vi "ClassPanel.vi"(8 "error in (no error)":errorcluster caption="entrée d'erreur (pas d'erreur)", 11 "DAQ6363.lvclass":refnum<class "DAQ6363.lvclass">) -> (0 "error out":errorcluster caption="sortie d'erreur", 3 "DAQ6363.lvclass Out":refnum<class "DAQ6363.lvclass">)   [LabVIEW 2019, in "DAQ6363.lvclass"]
uses:
  DAQ6363.lvclass
  C:/Programmes Labview/LabScanV1A/DevicesClass/BaseDevice/BaseDevice.lvclass
  BaseDevice/ClassQueueMess.ctl
  BaseDevice/BaseDevice.lvclass/BaseDevice.ctl
  DAQ6363.lvclass/DAQ6363.ctl
  BaseDevice/Accessor/SetShowInstrNm.vi
  BaseDevice/Accessor/GetClassEvent.vi
  <vilib>/DAQmx/create/channels.llb/DAQmx Create Channel (CI-Count Edges).vi
  <resource>/objmgr/daqmx.rc
panel:
  out "RtAvg Data":i32[][](array[numeric]) format="%.2f"
  out "Rate Data":i32[][](array[numeric])
  out "ClearRef":refnum<vi>
  out "Graph":refnum<vi>
  out "Dat":refnum<vi>
  out "ViRef":refnum<vi>
  out "Avg ref":refnum<vi>
  out "RtGrphAct":bool
  out "DeltaCh2(ms)":u32
  out "DeltaCh1(ms)":u32
  out "ReadCnts":bool
  out "Ch2CntTask":refnum<k21>
  out "Ch1CntTask":refnum<k21>
  in  "DAQ6363 Tabs":enum32{"Main", "Advanced"}(tab)
  in  "AcqTime":dbl=60.0 caption="Acqu. Time (ms)" min=0.1 step=0.1 format="%#.1f"
  out "TimeLeft":dbl caption="Time left(ms)" format="%<%H:%M:%S%1u>t"
  in  "ReadCont":bool caption="Read\nCont."
  out "Count Rates":u32[](array[numeric]) format="%#.0f"
  in  "ClearGrp":bool
  in  "Rate Graph":bool caption="Rate\nGraph"
  in  "Channel 1":bool
  in  "Channel 2":bool
  out "Jitter":bool
  in  "edge 2":i32(ring)=10280 caption="Ch2 Edge" items=["Rising"=10280, "Falling"=10171]
  in  "Ch2 Counter":tag="Dev1/ctr1"
  in  "Ch1 Counter":tag="Dev1/ctr0"
  in  "edge":i32(ring)=10280 caption="Ch1 Edge" items=["Rising"=10280, "Falling"=10171]
  in  "Ch1 Input":tag="/Dev1/PFI10"
  in  "Ch2 Input":tag="PFI8"
  in  "MainProgQ":refnum<queue>
  in  "MainProgQEvent":refnum<user-event>
  in  "Acq":bool
  in  "Stop":bool
  out "Init Program":bool
  # "DAQ6363"
  # "this MUST labeled with class name"
  # "this MUST be present and labeled \"Stop\" and \"Acq\""
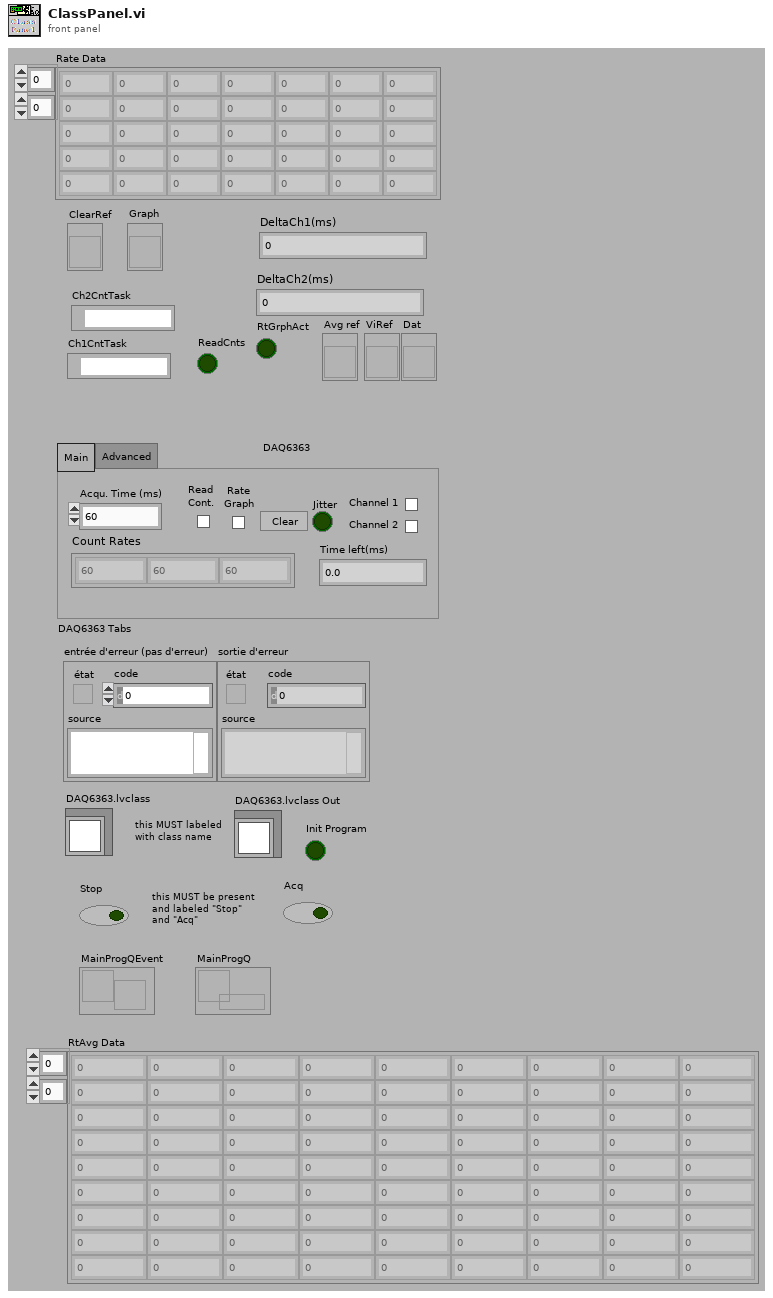
[diagram p1: front panel]
types:
  T1 = enum32{"Invalid", "Standard", "Closed", "Hidden", "Minimized", "Maximized"}
  T2 = cluster{dbl, "Refresh(ms)":u32, "Rate Data Out":i32[][]}
  T3 = typedef "ClassQueueMess.ctl" = u16
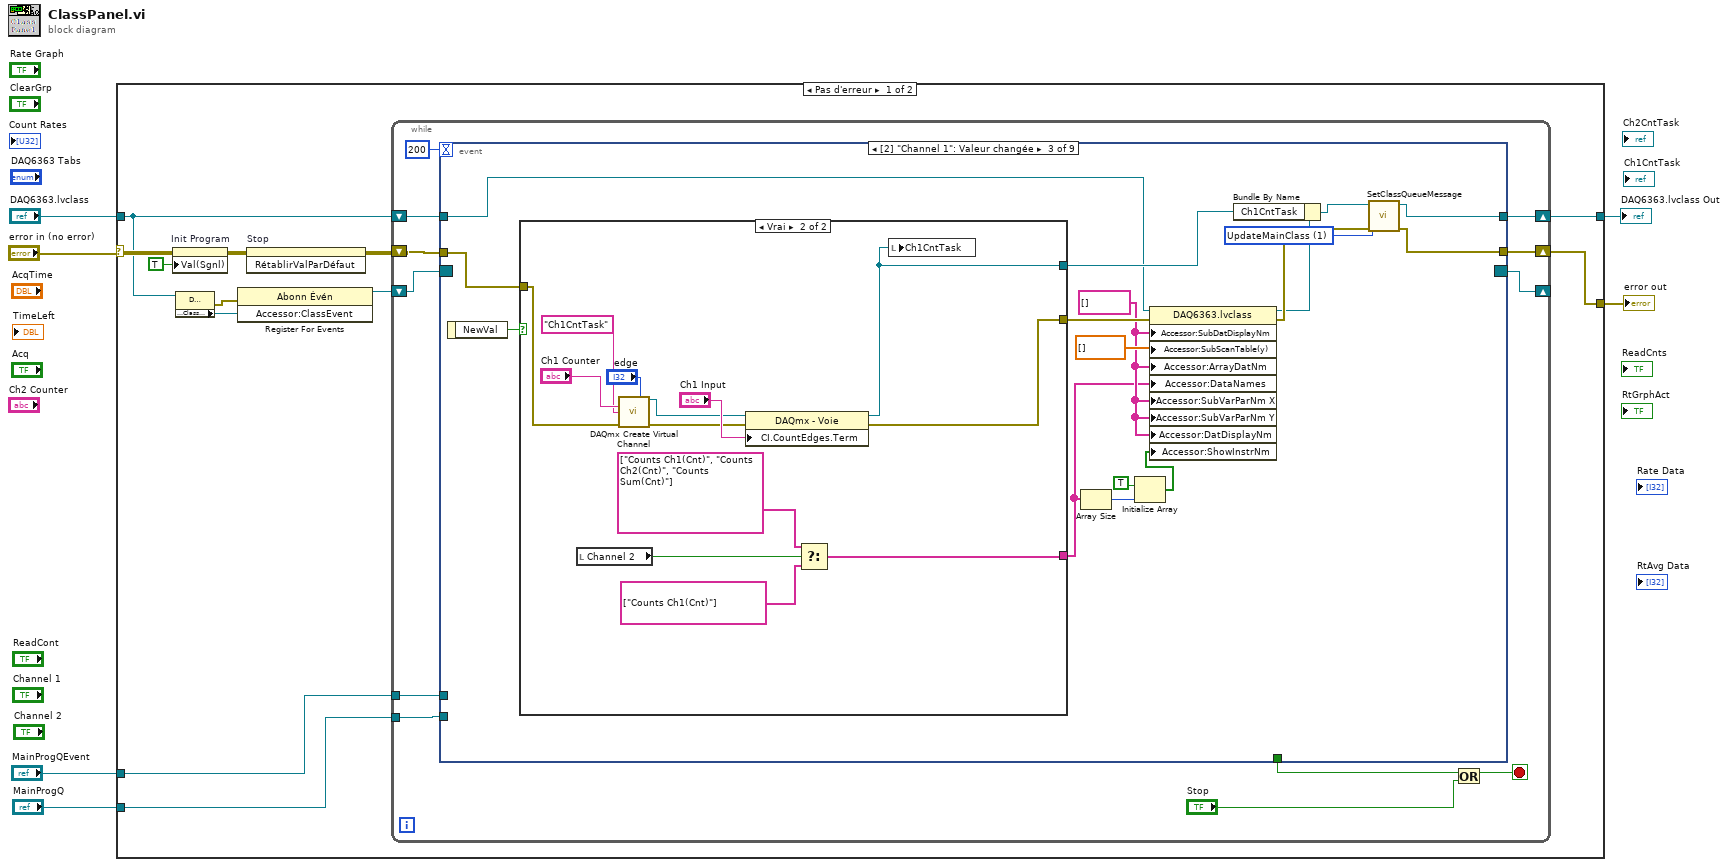
[diagram p0: block diagram]
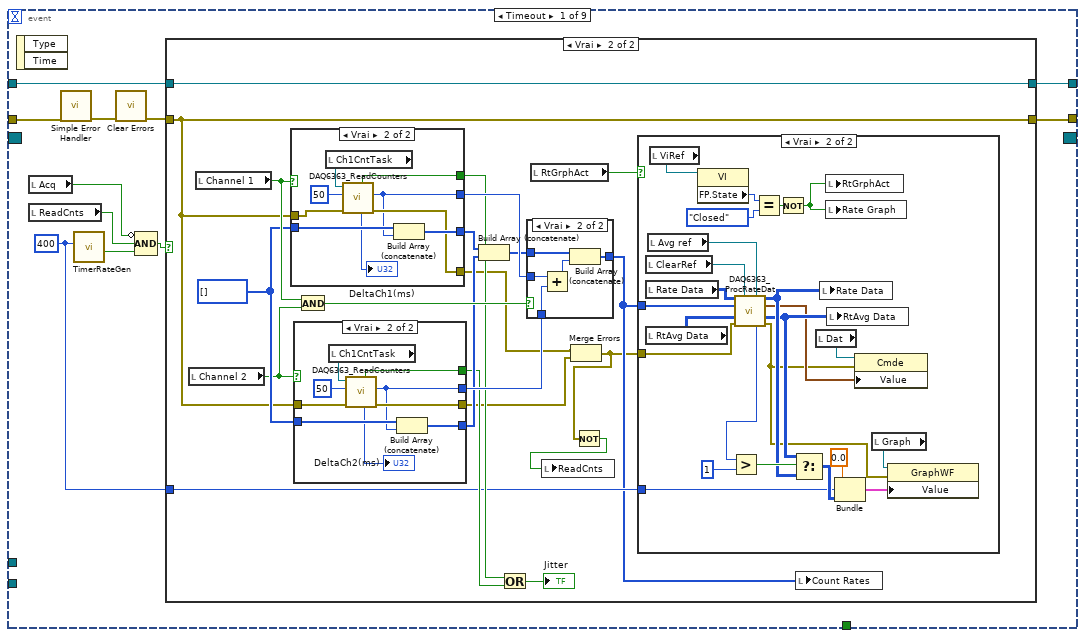
[diagram p2: hidden frame]
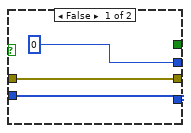
[diagram p5: hidden frame]
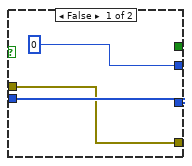
[diagram p7: hidden frame]
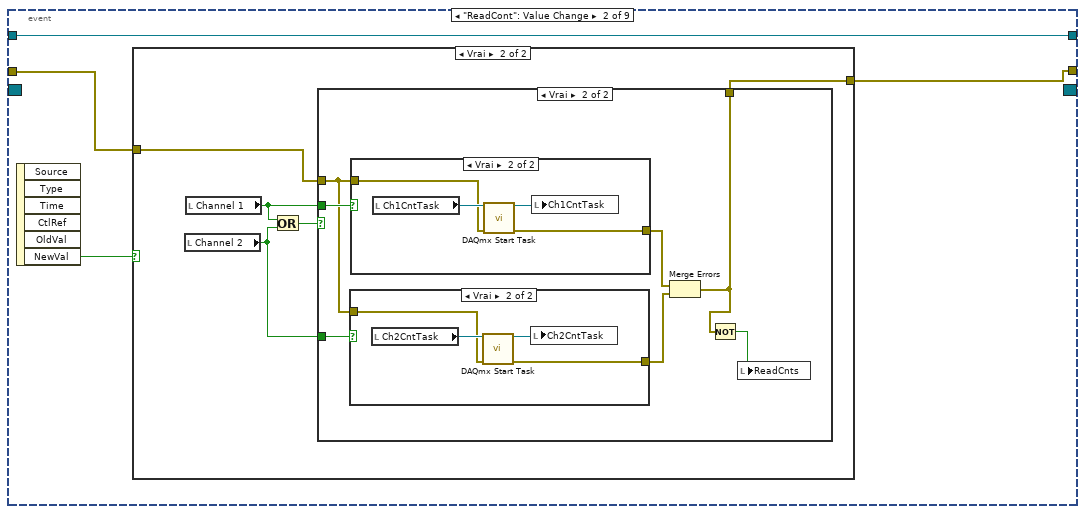
[diagram p8: hidden frame]
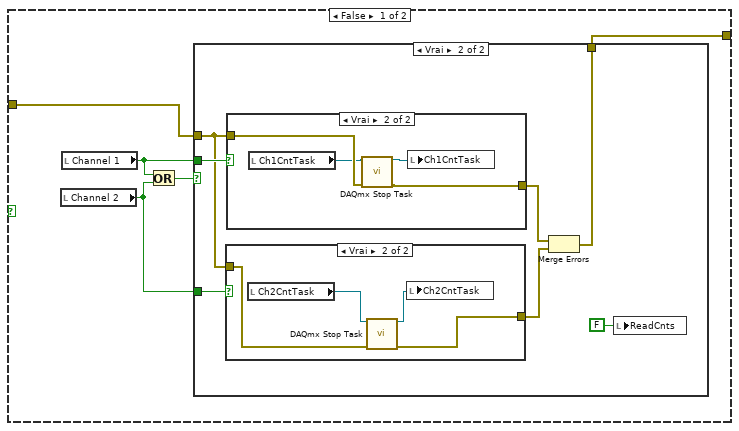
[diagram p9: hidden frame]
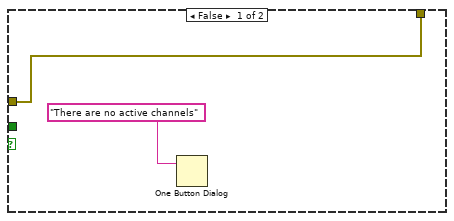
[diagram p13: hidden frame]
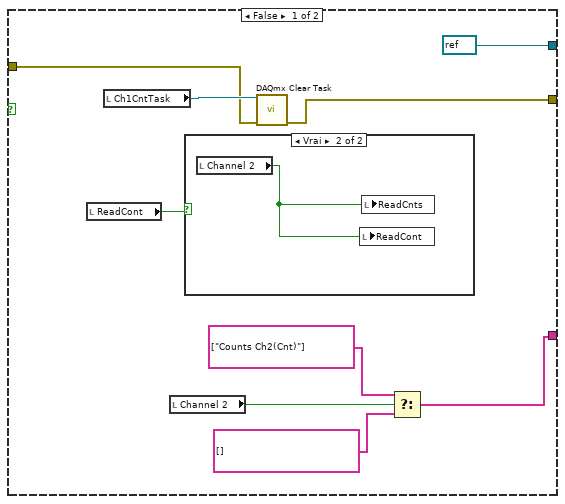
[diagram p16: hidden frame]
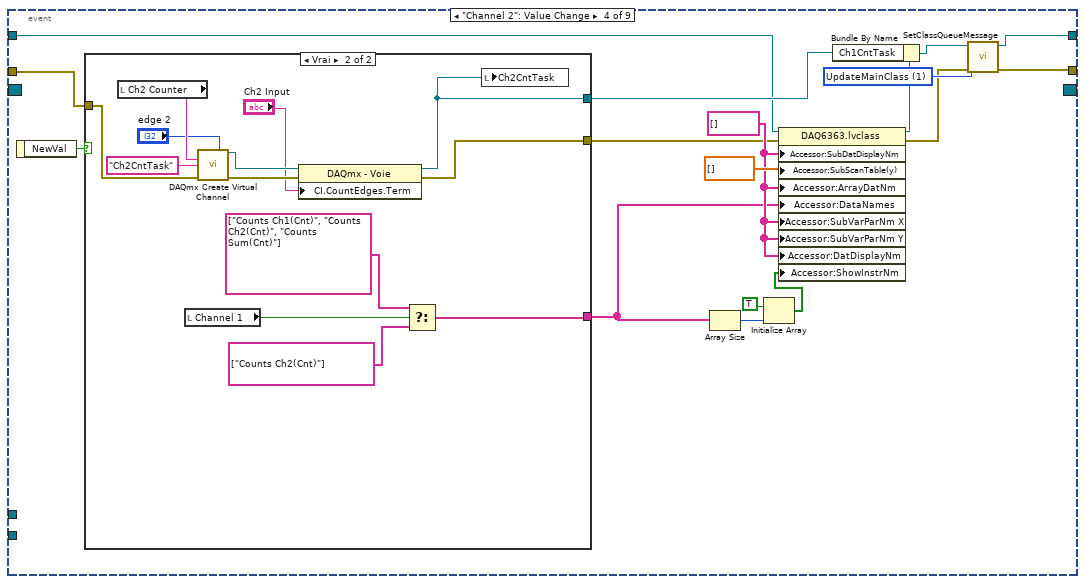
[diagram p18: hidden frame]
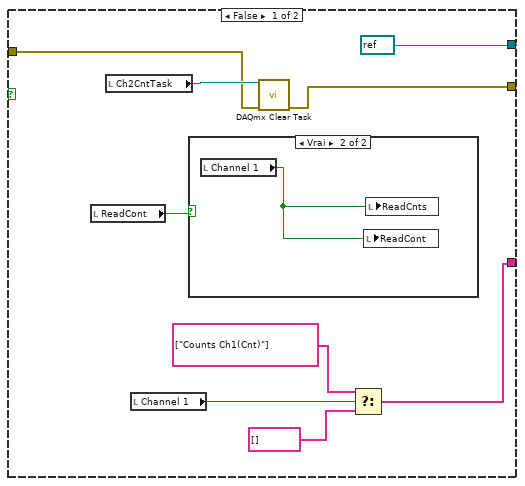
[diagram p19: hidden frame]
diagram:
  n1 = case shown="Pas d'erreur" "error in (no error)" {
    selector: "error in (no error)" -> [w15 w329]
    tunnel: [w18 w329] -> w5
    tunnel: "DAQ6363.lvclass" -> [w10 w328]
    tunnel: [w16 w328] -> w3
    tunnel: "MainProgQEvent" -> [w8 _]
    tunnel: "MainProgQ" -> [w7 _]
    frame No Error {
      n2 = property on="Init Program" class="Bool (strict)"(error in=w15, "Val(Sgnl)"=TRUE ("Valeur (Signalisation)")) -> (error out=w14:errorcluster)  [unwired: 1 in, 1 out]
      n3 = property class="DAQ6363.lvclass"(reference=w10) -> (error out=w12:errorcluster, "Accessor:ClassEvent"=w11:refnum<user-event>)  [unwired: 1 in, 1 out]
      n4 = register-events(error in=w12, w11) -> (reference out=w9:refnum<event-registration>)  [unwired: 1 in, 1 out]
      n5 = invoke on="Stop" class="Bool (strict)" method="RétablirValParDéfaut"(error in=w14) -> (error out=w13:errorcluster)  [unwired: 2 in, 2 out]
      n6 = while {
        shift-right: [w28] -> w18
        shift-left: w13 -> [w29]
        shift-right: [w25] -> w16
        shift-left: w10 -> [w27]
        shift-right: [w21] -> _
        shift-left: w9 -> [w22]
        tunnel: w8 -> [w20]
        tunnel: w7 -> [w19]
        stop <- w24 stop-if-true
        n7 = event shown="[2] \"Channel 1\": Valeur changée" {
          selector: w22 -> [_ _ _ _ _ _ _ _ _]
          dyn-events: [_ _ _ _ _ _ _ _ _] -> w21
          timeout: 200 -> [_ _ _ _ _ _ _ _ _]
          tunnel: w29 -> [w41 w121 w185 w225 w251 w267 w285 w314 w321]
          tunnel: [w32 w119 w180 w221 w250 w266 w279 w314 w320] -> w28
          tunnel: w27 -> [w39 w122 w179 w214 w252 w265 w286 w313 w318]
          tunnel: [_ _ _ _ _ _ _ TRUE FALSE] -> w26
          tunnel: [w40 w122 w182 w222 w252 w265 w278 w313 w317] -> w25
          tunnel: w20 -> [_ _ _ _ _ _ w277 _ _]
          tunnel: w19 -> [_ _ _ _ _ _ w276 _ _]
          event Timeout {
            w31 = u32 400 ("Refresh(ms)")
            n8 = event-data() -> ()  [unwired: 1 in, 2 out]
            n9 = local read "Acq"() -> (w35:bool)
            n10 = local read "ReadCnts"() -> (w36:bool)
            n11 = call <vilib>:"Simple Error Handler.vi"("error in (no error)"=w41) -> ("error out"=w34:errorcluster)  [unwired: 4 in, 4 out]
            n12 = call <userlib>:"TimerRateGen.vi"("Refresh(ms)"=w31) -> ("updated?"=w38:bool)  [unwired: 8 in, 2 out]
            n13 = call <vilib>:"Clear Errors.vi"("error in (no error)"=w34) -> ("error out"=w33:errorcluster)  [unwired: 5 in, 1 out]
            n14 = Compound Arithmetic op=AND(invert w35, w36, w38) -> (w37:bool)
            n15 = case shown="Vrai" w37 {
              tunnel: w33 -> [w42 w57]
              tunnel: [w42 w57] -> w32
              tunnel: [w43 w64] -> w40
              tunnel: w39 -> [w43 w64]
              tunnel: w31 -> [_ w49]
              frame False {
              }
              frame True {
                w58 = u32[] []
                n16 = local read "Channel 2"() -> (w56:bool)
                n17 = local read "Channel 1"() -> (w62:bool)
                n18 = case shown="Vrai" w62 {
                  tunnel: w57 -> [w107 w115]
                  tunnel: [u32 0 w111] -> w63
                  tunnel: [w107 w113] -> w46
                  tunnel: w58 -> [w109 w118]
                  tunnel: [w109 w117] -> w61
                  tunnel: [_ w110] -> w53
                  frame False {
                  }
                  frame True {
                    n19 = local read "Ch1CntTask"() -> (w116:refnum<k21>)
                    n20 = call <userlib>:"DAQ6363_ReadCounters.vi"("ErrIn(No Err)"=w115, "Count Period (ms)"=u32 50, "CntTask"=w116) -> ("ErrOut"=w113:errorcluster, "Counts/s"=w111:u32, "Period(ms)"=→"DeltaCh1(ms)":u32, "Jitter Warning"=w110:bool)  [unwired: 3 in, 2 out]
                    n21 = Build Array (concatenate)(w118, w111) -> (w117:u32[])
                  }
                }
                n22 = case shown="Vrai" w56 {
                  tunnel: w57 -> [w89 w97]
                  tunnel: [u32 0 w94] -> w55
                  tunnel: [w89 w95] -> w47
                  tunnel: w58 -> [w91 w100]
                  tunnel: [w91 w99] -> w54
                  tunnel: [_ w93] -> w52
                  frame False {
                  }
                  frame True {
                    n23 = local read "Ch1CntTask"() -> (w98:refnum<k21>)
                    n24 = call <userlib>:"DAQ6363_ReadCounters.vi"("ErrIn(No Err)"=w97, "Count Period (ms)"=u32 50, "CntTask"=w98) -> ("ErrOut"=w95:errorcluster, "Counts/s"=w94:u32, "Period(ms)"=→"DeltaCh2(ms)":u32, "Jitter Warning"=w93:bool)  [unwired: 3 in, 2 out]
                    n25 = Build Array (concatenate)(w100, w94) -> (w99:u32[])
                  }
                }
                n26 = And(x=w62, y=w56) -> (x .and. y?=w60:bool)
                n27 = Build Array (concatenate)(w61, w54) -> (w59:u32[])
                n28 = Or(x=w53, y=w52) -> (x .or. y?=→"Jitter":bool)
                n29 = case shown="Vrai" w60 {
                  tunnel: w63 -> [_ w106]
                  tunnel: w55 -> [_ w105]
                  tunnel: w59 -> [w101 w103]
                  tunnel: [w101 w102] -> w48
                  frame False {
                  }
                  frame True {
                    n30 = Add(x=w106, y=w105) -> (x+y=w104:u32)
                    n31 = Build Array (concatenate)(w103, w104) -> (w102:u32[])
                  }
                }
                n32 = local read "RtGrphAct"() -> (w50:bool)
                n33 = Merge Errors(w46, w47) -> (w45:errorcluster)
                n34 = Not(x=w45) -> (.not. x?=w44:bool)
                n35 = local write "ReadCnts"(w44) -> ()
                n36 = case shown="Vrai" w50 {
                  tunnel: w49 -> [_ w73]
                  tunnel: w48 -> [_ w70]
                  tunnel: w45 -> [_ w68]
                  frame False {
                  }
                  frame True {
                    n37 = local read "ClearRef"() -> (w83:refnum<vi>)
                    n38 = local read "Rate Data"() -> (w66:i32[][])
                    n39 = local read "RtAvg Data"() -> (w65:i32[][])
                    n40 = local read "Avg ref"() -> (w82:refnum<vi>)
                    n41 = local read "ViRef"() -> (w88:refnum<vi>)
                    n42 = property class="VI"(reference=w88) -> ("FP.State"=w86:T1)  [unwired: 1 in, 2 out]
                    n43 = call <userlib>:"DAQ6363_ProcRateDat.vi"("Rate Data"=w66, "ClearRef"=w83, "Avg ref"=w82, "Count Rates"=w70, "RateAvg Data"=w65, "error in (no error)"=w68) -> ("Rate Data Out"=w76:i32[][], "Data"=w71:cluster{dbl, dbl, dbl, dbl}[], "RateAvg Data Out"=w75:i32[][], "Avg Val Out"=w77:i32, "error out"=w69:errorcluster)  [unwired: 4 in, 1 out]
                    n44 = Greater?(x=w77, y=1) -> (0:w79:bool)
                    n45 = Equal?(x=w86, y=T1."Closed") -> (x = y?=w87:bool)
                    n46 = Not(x=w87) -> (.not. x?=w84:bool)
                    n47 = Select(t=w75, s=w79, f=w76) -> (s? t:f=w78:i32[][])
                    n48 = local read "Dat"() -> (w67:refnum<vi>)
                    n49 = local write "Rate Data"(w76) -> ()
                    n50 = local write "RtGrphAct"(w84) -> ()
                    n51 = local write "Rate Graph"(w84) -> ()
                    n52 = local write "RtAvg Data"(w75) -> ()
                    n53 = Bundle(0.0, "Refresh(ms)"=w73, "Rate Data Out"=w78) -> (w74:T2)  [unwired: 1 in]
                    n54 = property class="Cmde"(reference=w67, error in=w69, "Value"=w71) -> ()  [unwired: 2 out]
                    n55 = local read "Graph"() -> (w72:refnum<vi>)
                    n56 = property class="GraphWF"(reference=w72, error in=w69, "Value"=w74) -> ()  [unwired: 2 out]
                  }
                }
                n57 = local write "Count Rates"(w48) -> ()
              }
            }
          }
          event "ReadCont": Value Change {
            n58 = event-data() -> ("NewVal"=w120:bool)  [unwired: 1 in, 5 out]
            n59 = case shown="Vrai" w120 {
              tunnel: w121 -> [w125 w148]
              tunnel: [w123 w146] -> w119
              frame False {
                n60 = local read "Channel 2"() -> (w124:bool)
                n61 = local read "Channel 1"() -> (w126:bool)
                n62 = Or(x=w126, y=w124) -> (x .or. y?=w127:bool)
                n63 = case shown="Vrai" w127 {
                  tunnel: w126 -> [_ w135]
                  tunnel: w125 -> [w128 w134]
                  tunnel: w124 -> [_ w131]
                  tunnel: [w128 w130] -> w123
                  frame False {
                  }
                  frame True {
                    n64 = case shown="Vrai" w131 {
                      tunnel: w134 -> [w136 w140]
                      tunnel: [w136 w138] -> w132
                      frame False {
                      }
                      frame True {
                        n65 = local read "Ch2CntTask"() -> (w139:refnum<k21>)
                        n66 = call <vilib>:"DAQmx Stop Task.vi"("task/channels in"=w139, "error in"=w140) -> ("task out"=w137:refnum<k21>, "error out"=w138:errorcluster)  [unwired: 12 in]
                        n67 = local write "Ch2CntTask"(w137) -> ()
                      }
                    }
                    n68 = case shown="Vrai" w135 {
                      tunnel: w134 -> [w141 w144]
                      tunnel: [w141 w145] -> w133
                      frame False {
                      }
                      frame True {
                        n69 = local read "Ch1CntTask"() -> (w143:refnum<k21>)
                        n70 = call <vilib>:"DAQmx Stop Task.vi"("task/channels in"=w143, "error in"=w144) -> ("task out"=w142:refnum<k21>, "error out"=w145:errorcluster)  [unwired: 12 in]
                        n71 = local write "Ch1CntTask"(w142) -> ()
                      }
                    }
                    n72 = Merge Errors(w133, w132) -> (w130:errorcluster)
                    n73 = local write "ReadCnts"(FALSE ("ReadCnts")) -> ()
                  }
                }
              }
              frame True {
                n74 = local read "Channel 2"() -> (w147:bool)
                n75 = local read "Channel 1"() -> (w149:bool)
                n76 = Or(x=w149, y=w147) -> (x .or. y?=w150:bool)
                n77 = case shown="Vrai" w150 {
                  tunnel: w149 -> [_ w159]
                  tunnel: w148 -> [w151 w158]
                  tunnel: w147 -> [_ w155]
                  tunnel: [w151 w154] -> w146
                  frame False {
                    n78 = One Button Dialog(message="There are no active channels") -> ()  [unwired: 1 in, 1 out]
                  }
                  frame True {
                    n79 = case shown="Vrai" w155 {
                      tunnel: w158 -> [w160 w163]
                      tunnel: [w160 w161] -> w156
                      frame False {
                      }
                      frame True {
                        n80 = local read "Ch2CntTask"() -> (w164:refnum<k21>)
                        n81 = call <vilib>:"DAQmx Start Task.vi"("task/channels in"=w164, "error in"=w163) -> ("task out"=w162:refnum<k21>, "error out"=w161:errorcluster)  [unwired: 12 in]
                        n82 = local write "Ch2CntTask"(w162) -> ()
                      }
                    }
                    n83 = case shown="Vrai" w159 {
                      tunnel: w158 -> [w165 w168]
                      tunnel: [w165 w166] -> w157
                      frame False {
                      }
                      frame True {
                        n84 = local read "Ch1CntTask"() -> (w169:refnum<k21>)
                        n85 = call <vilib>:"DAQmx Start Task.vi"("task/channels in"=w169, "error in"=w168) -> ("task out"=w167:refnum<k21>, "error out"=w166:errorcluster)  [unwired: 12 in]
                        n86 = local write "Ch1CntTask"(w167) -> ()
                      }
                    }
                    n87 = Merge Errors(w157, w156) -> (w154:errorcluster)
                    n88 = Not(x=w154) -> (.not. x?=w153:bool)
                    n89 = local write "ReadCnts"(w153) -> ()
                  }
                }
              }
            }
          }
          event "Channel 1": Value Change {
            w175 = string[] [] ("SubDatDisplayNm")
            w181 = T3 1 items=["UpdateClassData", "UpdateMainClass", "UpdateDataBind", "ReInitDevice", "Custom", "ClosePan"] ("Menu déroulant")
            n90 = event-data() -> ("NewVal"=w186:bool)  [unwired: 1 in]
            n91 = case shown="Vrai" w186 {
              tunnel: w185 -> [w194 w207]
              tunnel: [w193 w202] -> w176
              tunnel: [refnum<k21> refnum ("task out") w203] -> w184
              tunnel: [w187 w198] -> w171
              frame False {
                n92 = local read "ReadCont"() -> (w192:bool)
                n93 = local read "Ch1CntTask"() -> (w195:refnum<k21>)
                n94 = local read "Channel 2"() -> (w190:bool)
                n95 = case shown="Vrai" w192 {
                  frame False {
                  }
                  frame True {
                    n96 = local read "Channel 2"() -> (w196:bool)
                    n97 = local write "ReadCont"(w196) -> ()
                    n98 = local write "ReadCnts"(w196) -> ()
                  }
                }
                n99 = call <vilib>:"DAQmx Clear Task.vi"("task in"=w195, "error in"=w194) -> ("error out"=w193:errorcluster)  [unwired: 13 in]
                n100 = Select(t=string[] ["Counts Ch2(Cnt)"], s=w190, f=string[] []) -> (s? t:f=w187:string[])
              }
              frame True {
                n101 = local read "Channel 2"() -> (w201:bool)
                n102 = call-poly <vilib>:"DAQmx Create Virtual Channel.vi"("edge"="edge", "counter"="Ch1 Counter", "name to assign"="Ch1CntTask", "error in"=w207) -> ("task out"=w205:refnum<k21>, "error out"=w204:errorcluster)  [unwired: 10 in]
                n103 = property class="DAQmx - Voie"(reference=w205, error in=w204, "CI.CountEdges.Term"="Ch1 Input") -> (reference out=w203:refnum<k21>, error out=w202:errorcluster)
                n104 = Select(t=string[] ["Counts Ch1(Cnt)", "Counts Ch2(Cnt)", "Counts Sum(Cnt)"], s=w201, f=string[] ["Counts Ch1(Cnt)"]) -> (s? t:f=w198:string[])
                n105 = local write "Ch1CntTask"(w203) -> ()
              }
            }
            n106 = Array Size(array=w171) -> (size(s)=w174:i32)
            n107 = Initialize Array(TRUE, w174) -> (w172:bool[])
            n108 = property class="DAQ6363.lvclass"(reference=w179, error in=w176, "Accessor:SubDatDisplayNm"=w175, "Accessor:SubScanTable(y)"=dbl[] [] ("SubScanTable(y)"), "Accessor:ArrayDatNm"=w175, "Accessor:DataNames"=w171, "Accessor:SubVarParNm X"=w175, "Accessor:SubVarParNm Y"=w175, "Accessor:DatDisplayNm"=w175, "Accessor:ShowInstrNm"=w172) -> (reference out=w170:refnum<class "DAQ6363.lvclass">, error out=w178:errorcluster)
            n109 = Bundle By Name(cluster=w170, "Ch1CntTask"=w184) -> (w183:refnum<class "DAQ6363.lvclass">)
            n110 = call-dynamic "SetClassQueueMessage.vi"("ErrorIn(No Error)"=w178, "Menu déroulant"=w181, "DefaultDev.lvclass"=w183) -> ("sortie d'erreur"=w180:errorcluster, "DefaultDev.lvclass Out"=w182:refnum<class "DAQ6363.lvclass">)  [unwired: 7 in]
          }
          event "Channel 2": Value Change {
            w218 = string[] [] ("SubDatDisplayNm")
            w223 = T3 1 items=["UpdateClassData", "UpdateMainClass", "UpdateDataBind", "ReInitDevice", "Custom", "ClosePan"] ("Menu déroulant")
            n111 = event-data() -> ("NewVal"=w226:bool)  [unwired: 1 in]
            n112 = case shown="Vrai" w226 {
              tunnel: w225 -> [w234 w249]
              tunnel: [w233 w245] -> w212
              tunnel: [refnum<k21> refnum ("Ch2CntTask") w242] -> w220
              tunnel: [w228 w238] -> w210
              frame False {
                n113 = local read "ReadCont"() -> (w232:bool)
                n114 = local read "Ch2CntTask"() -> (w235:refnum<k21>)
                n115 = local read "Channel 1"() -> (w230:bool)
                n116 = case shown="Vrai" w232 {
                  frame False {
                  }
                  frame True {
                    n117 = local read "Channel 1"() -> (w236:bool)
                    n118 = local write "ReadCont"(w236) -> ()
                    n119 = local write "ReadCnts"(w236) -> ()
                  }
                }
                n120 = call <vilib>:"DAQmx Clear Task.vi"("task in"=w235, "error in"=w234) -> ("error out"=w233:errorcluster)  [unwired: 13 in]
                n121 = Select(t=string[] ["Counts Ch1(Cnt)"], s=w230, f=string[] [] ("cas faux")) -> (s? t:f=w228:string[])
              }
              frame True {
                n122 = local read "Ch2 Counter"() -> (w248:tag)
                n123 = local read "Channel 1"() -> (w241:bool)
                n124 = call-poly <vilib>:"DAQmx Create Virtual Channel.vi"("edge"="edge 2", "counter"=w248, "name to assign"="Ch2CntTask", "error in"=w249) -> ("task out"=w244:refnum<k21>, "error out"=w246:errorcluster)  [unwired: 10 in]
                n125 = property class="DAQmx - Voie"(reference=w244, error in=w246, "CI.CountEdges.Term"="Ch2 Input") -> (reference out=w242:refnum<k21>, error out=w245:errorcluster)
                n126 = Select(t=string[] ["Counts Ch1(Cnt)", "Counts Ch2(Cnt)", "Counts Sum(Cnt)"], s=w241, f=string[] ["Counts Ch2(Cnt)"]) -> (s? t:f=w238:string[])
                n127 = local write "Ch2CntTask"(w242) -> ()
              }
            }
            n128 = Array Size(array=w210) -> (size(s)=w217:i32)
            n129 = Initialize Array(TRUE, w217) -> (w215:bool[])
            n130 = property class="DAQ6363.lvclass"(reference=w214, error in=w212, "Accessor:SubDatDisplayNm"=w218, "Accessor:SubScanTable(y)"=dbl[] [] ("SubScanTable(y)"), "Accessor:ArrayDatNm"=w218, "Accessor:DataNames"=w210, "Accessor:SubVarParNm X"=w218, "Accessor:SubVarParNm Y"=w218, "Accessor:DatDisplayNm"=w218, "Accessor:ShowInstrNm"=w215) -> (reference out=w213:refnum<class "DAQ6363.lvclass">, error out=w211:errorcluster)
            n131 = Bundle By Name(cluster=w213, "Ch1CntTask"=w220) -> (w224:refnum<class "DAQ6363.lvclass">)
            n132 = call-dynamic "SetClassQueueMessage.vi"("ErrorIn(No Error)"=w211, "Menu déroulant"=w223, "DefaultDev.lvclass"=w224) -> ("sortie d'erreur"=w221:errorcluster, "DefaultDev.lvclass Out"=w222:refnum<class "DAQ6363.lvclass">)  [unwired: 7 in]
          }
          event "Rate Graph": Value Change {
            n133 = event-data() -> ("NewVal"=w253:bool)  [unwired: 1 in, 5 out]
            n134 = case shown="Vrai" w253 {
              selector: w253 -> [w254 _]
              tunnel: w251 -> [w255 w259]
              tunnel: [w255 w257] -> w250
              frame False {
                n135 = local write "RtGrphAct"(w254) -> ()
              }
              frame True {
                n136 = call <userlib>:"DAQ6363_LoadHistGraph.vi"("ErrIn(No Err)"=w259, "Rate Mode"=TRUE) -> ("ErrOut"=w257:errorcluster, "Graph"=→"Graph":refnum<vi>, "Dat"=→"Dat":refnum<vi>, "ViRef"=→"ViRef":refnum<vi>, "Avg ref"=→"Avg ref":refnum<vi>, "ClearRef"=→"ClearRef":refnum<vi>)  [unwired: 3 in, 1 out]
                n137 = Not(x=w257) -> (.not. x?=w256:bool)
                n138 = local write "RtGrphAct"(w256) -> ()
              }
            }
          }
          event "ClearGrp": Value Change {
            n139 = event-data() -> ("NewVal"=w268:bool)  [unwired: 1 in, 5 out]
            n140 = Wait (ms)(milliseconds to wait=u32 400 ("attente (ms)")) -> ()  [unwired: 1 out]
            n141 = case shown="Vrai" w268 {
              tunnel: w267 -> [w270 w272]
              tunnel: [w270 w271] -> w266
              frame False {
              }
              frame True {
                n142 = local read "ClearRef"() -> (w274:refnum<vi>)
                n143 = call <userlib>:"WritebyWeakRefBool.vi"("error in"=w272, "Valeur"=TRUE, "Control Ref"=w274) -> ("error out"=w271:errorcluster)  [unwired: 8 in]
                n144 = local write "ClearGrp"(FALSE ("ClearGrp")) -> ()
              }
            }
          }
          event User Event {
            n145 = event-data() -> ("queue out"=w283:refnum<queue>)  [unwired: 1 in, 3 out]
            n146 = Dequeue Element(queue=w283) -> (element=w284:cluster{"Message":string, "Data":variant, i32})  [unwired: 2 in, 3 out]
            n147 = Unbundle(w284) -> ("Message"=w282:string, "Data"=w281:variant, w280:i32)
            n148 = case shown="\"UpdateClassData\"" w282 {
              tunnel: w285 -> [w288 w292 w294 w298 w302 w305]
              tunnel: w281 -> [_ w291 w297 _ _ _]
              tunnel: w286 -> [w287 w290 w296 w299 w303 w308]
              tunnel: [w287 w289 w295 w299 w303 w308] -> w278
              tunnel: [w288 w292 w293 w298 w302 w304] -> w279
              tunnel: w280 -> [_ _ _ _ _ _]
              tunnel: w277 -> [_ _ _ _ _ w307]
              tunnel: w276 -> [_ _ _ _ _ w306]
              frame Default {
              }
              frame "UpdateClassData" {
                n149 = Variant To Data(type=w290, Variant=w291) -> (data=w289:refnum<class "DAQ6363.lvclass">)  [unwired: 1 in, 1 out]
              }
              frame "UpdateDataBind" {
                n150 = Variant To Data(error in=w294, type=w296, Variant=w297) -> (data=w295:refnum<class "DAQ6363.lvclass">, error out=w293:errorcluster)
              }
              frame "MeasDone" {
              }
              frame "ShowDiag" {
                n151 = control-ref of="This VI"() -> (w301:refnum<vi>)
                n152 = call <userlib>:"AnimExecGen.vi"("Animer l'exécution ?"=TRUE, "ViRef"=w301) -> ()  [unwired: 9 in, 1 out]
              }
              frame "UpdateMainClass" {
                n153 = Bundle By Name(cluster=cluster{"Message":string, "Data":variant, i32} {"Message"="", "Data"=variant, 0} ("élément"), "Data"=w308) -> (w309:cluster{"Message":string, "Data":variant, i32})
                n154 = Enqueue Element(queue=w306, element=w309, error in (no error)=w305) -> (queue out=w312:refnum<queue>, error out=w311:errorcluster)  [unwired: 1 in, 1 out]
                n155 = Generate User Event(user event=w307, event data cluster=w312, error in=w311) -> (error out=w304:errorcluster)  [unwired: 1 in, 1 out]
              }
            }
          }
          event Panel Close? {
            n156 = event-data() -> ()  [unwired: 1 in, 1 out]
            n157 = event-data("Discard?"=FALSE ("Rejeter ?")) -> ()  [unwired: 1 in, 1 out]
          }
          event "Init Program": Value Change {
            n158 = event-data() -> ("NewVal"=w322:bool)  [unwired: 1 in]
            n159 = case shown="Vrai" w322 {
              tunnel: w321 -> [w324 w326]
              tunnel: [w324 w326] -> w320
              tunnel: [w323 w325] -> w317
              tunnel: w318 -> [w323 w325]
              frame False {
              }
              frame True {
                "Init Program" <- FALSE
              }
            }
          }
        }
        n160 = Or(x=w26, y="Stop") -> (x .or. y?=w24:bool)
      }
    }
    frame Error {
    }
  }
  "error out" <- w5
  "DAQ6363.lvclass Out" <- w3
